vi "Stage tester.vi"() -> ()   [LabVIEW 2017]
panel:
  in  "Z":dbl
  in  "Y":dbl
  in  "X":dbl
  in  "stop":bool
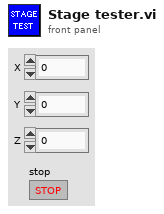
[diagram p1: front panel]
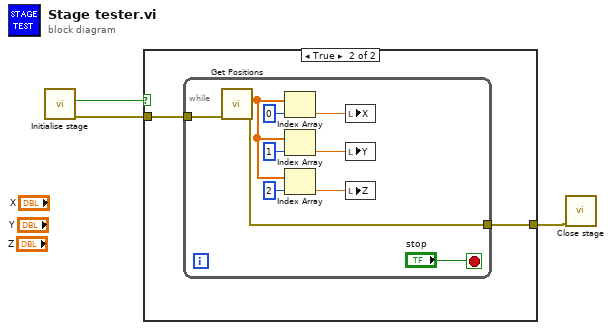
[diagram p0: block diagram]
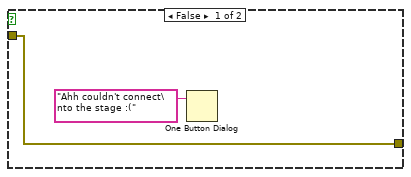
[diagram p2: hidden frame]
diagram:
  n1 = call "Initialise stage.vi"() -> ("error out"=w2:errorcluster, "Connected successfully"=w3:bool)  [unwired: 10 in]
  n2 = case shown="True" w3 {
    tunnel: w2 -> [w4 w7]
    tunnel: [w4 w6] -> w1
    frame False {
      n3 = One Button Dialog(message="Ahh couldn't connect\nto the stage :(") -> ()  [unwired: 1 in, 1 out]
    }
    frame True {
      n4 = while {
        tunnel: w7 -> [w16]
        tunnel: [w8] -> w6
        stop <- "stop" stop-if-true
        n5 = call "Get Positions.vi"("error in"=w16) -> ("error out"=w8:errorcluster, "Stage current position"=w9:dbl[])  [unwired: 9 in]
        n6 = Index Array(array=w9, index=0) -> (element=w14:dbl)
        n7 = Index Array(array=w9, index=1) -> (element=w13:dbl)
        n8 = Index Array(array=w9, index=2) -> (element=w10:dbl)
        n9 = local write "X"(w14) -> ()
        n10 = local write "Y"(w13) -> ()
        n11 = local write "Z"(w10) -> ()
      }
    }
  }
  n12 = call "Close stage.vi"("error in"=w1) -> ()  [unwired: 10 in, 1 out]
